vi "Model 3566-Error Handle.vi"(8 "error in":errorcluster, 11 "Respond In":string) -> (0 "error out":errorcluster, 3 "Respond Out":string)   [LabVIEW 2018]
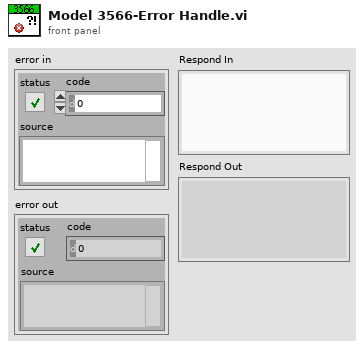
[diagram p1: front panel]
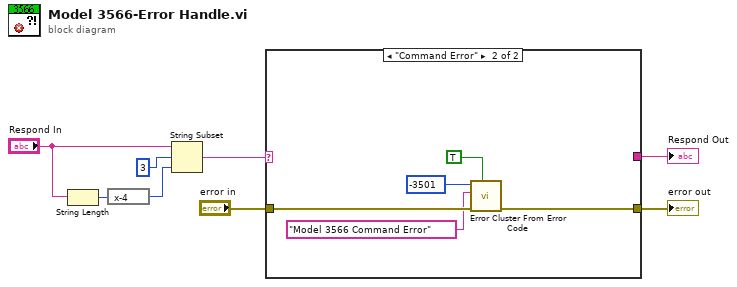
[diagram p0: block diagram]
diagram:
  n1 = String Length(string="Respond In") -> (length=w2:i32)
  n2 = expression code="x-4"(w2) -> (w1:i32)
  n3 = String Subset(string="Respond In", offset (0)=3, length (rest)=w1) -> (substring=w4:string)
  n4 = case shown="\"Command Error\"" w4 {
    selector: w4 -> [w10 _]
    tunnel: "error in" -> [w9 w15]
    tunnel: [w9 w14] -> w7
    tunnel: [w10 _] -> w6
    frame Default {
    }
    frame "Command Error" {
      n5 = call <vilib>:"Error Cluster From Error Code.vi"("show call chain? (False)"=TRUE, "error in (no error)"=w15, "error message (\"\")"="Model 3566 Command Error" ("error message (\"\")"), "error code (0)"=-3501) -> ("error out"=w14:errorcluster)  [unwired: 5 in]
    }
  }
  "error out" <- w7
  "Respond Out" <- w6
